vi "wait.vi"(0 "HGF_Rendezvous":refnum<class "HGF_Rendezvous.lvclass">, 3 "msTimeout (-1)":i32=-1, 5 "error in (no error)":errorcluster, 9 "ignore previous (F)":bool) -> (14 "dup HGF_Rendezvous":refnum<class "HGF_Rendezvous.lvclass">, 16 "Object":refnum<class>, 17 "timed out":bool, 19 "error out":errorcluster)   [LabVIEW 2014, in "HGF_BaseClasses.lvlib" / "HGF_Rendezvous.lvclass"]
doc: "Use this VI to wait on events.\n\n<b>Hint:</b> This is a shared reentrant VI."
uses:
  HGF_Rendezvous.lvclass
  HGF_Event/HGF_Event.lvclass
  HGF_Timing/HGF_Timing.lvclass
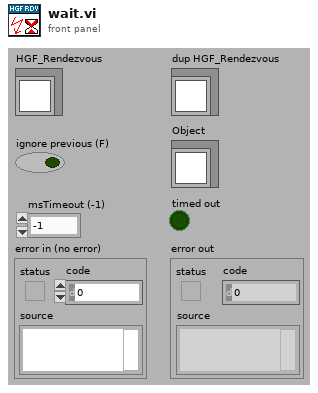
[diagram p1: front panel]
types:
  T1 = typedef "Rendezvous RefNum" = refnum<k1>
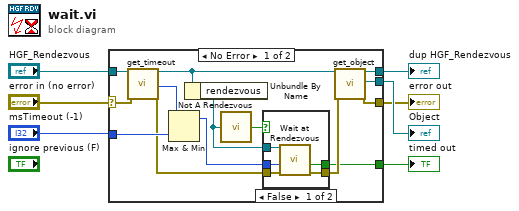
[diagram p0: block diagram]
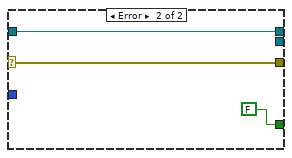
[diagram p3: hidden frame]
diagram:
  n1 = case shown="No Error" "error in (no error)" {
    selector: "error in (no error)" -> [w20 w29]
    tunnel: "HGF_Rendezvous" -> [w21 w30]
    tunnel: [w16 w30] -> w1
    tunnel: "msTimeout (-1)" -> [w18 _]
    tunnel: [w15 _] -> w3
    tunnel: [w10 FALSE ("timed out")] -> w4
    tunnel: [w14 w29] -> w2
    frame No Error {
      n2 = call "get_timeout.vi"("HGF_Event.lvclass in"=w21, "error in (no error)"=w20) -> ("HGF_Event.lvclass out"=w17:refnum<class "HGF_Rendezvous.lvclass">, "timeout"=w19:i32, "error out"=w12:errorcluster)  [unwired: 15 out]
      n3 = Max & Min(x=w19, y=w18) -> (max(x,y)=w13:i32)  [unwired: 1 out]
      n4 = Unbundle By Name(w17) -> ("rendezvous"=w9:T1)
      n5 = call <vilib>:"Not A Rendezvous.vi"("rendezvous"=w9) -> ("not a rendezvous"=w8:bool)
      n6 = case shown="False" w8 {
        tunnel: w13 -> [w26 _]
        tunnel: w12 -> [w25 w27]
        tunnel: [w24 w27] -> w11
        tunnel: [w23 _] -> w10
        tunnel: w9 -> [w22 _]
        frame False {
          n7 = call <vilib>:"Wait at Rendezvous.vi"("error in (no error)"=w25, "ms timeout (-1)"=w26, "rendezvous"=w22) -> ("error out"=w24:errorcluster, "timed out"=w23:bool)  [unwired: 3 out]
        }
        frame True {
        }
      }
      n8 = call "get_object.vi"("HGF_Timing.lvclass"=w17, "error in (no error)"=w11) -> ("dup HGF_Timing"=w16:refnum<class "HGF_Rendezvous.lvclass">, "object"=w15:refnum<class>, "error out"=w14:errorcluster)  [unwired: 15 out]
    }
    frame Error {
    }
  }
  "error out" <- w2
  "dup HGF_Rendezvous" <- w1
  "timed out" <- w4
  "Object" <- w3
